vi "Read Config_CSV_FilePath.vi"(8 "error in (no error)":errorcluster, 11 "MCLB_Template in":refnum<class "SCLB_Template.lvclass">) -> (0 "error out":errorcluster, 2 "Config_CSV_FilePath":path, 3 "MCLB_Template out":refnum<class "SCLB_Template.lvclass">)   [LabVIEW 2021, in "SCLB_Template.lvclass"]
uses:
  SCLB_Template.lvclass
  SCLB_Template.lvclass/SCLB_Template.ctl
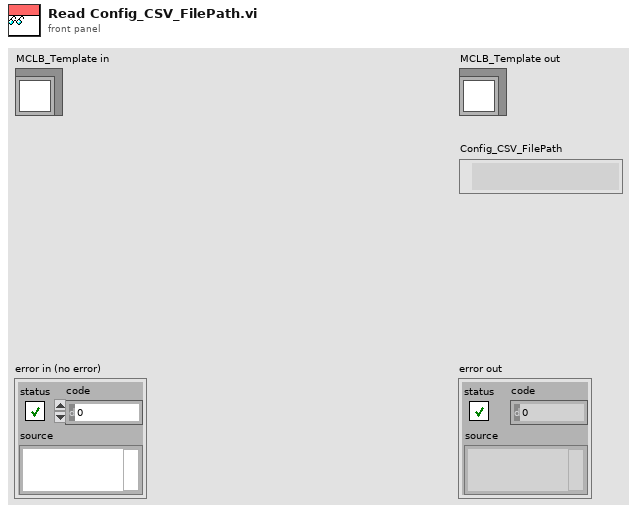
[diagram p1: front panel]
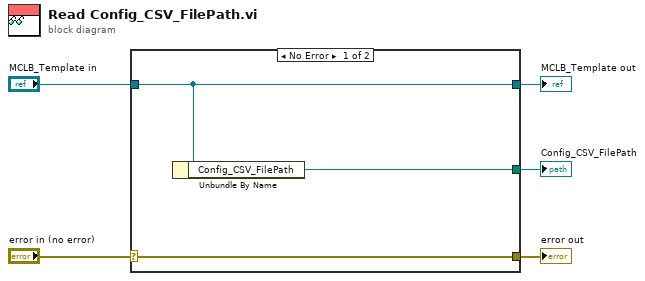
[diagram p0: block diagram]
diagram:
  n1 = case shown="No Error" "error in (no error)" {
    selector: "error in (no error)" -> [w8 w9]
    tunnel: [w8 w9] -> w4
    tunnel: [w7 w10] -> w2
    tunnel: "MCLB_Template in" -> [w7 w10]
    tunnel: [w6 _] -> w1
    frame No Error {
      n2 = Unbundle By Name(w7) -> ("Config_CSV_FilePath"=w6:path)
    }
    frame Error {
    }
  }
  "error out" <- w4
  "MCLB_Template out" <- w2
  "Config_CSV_FilePath" <- w1
